vi "Atheros Tx CAL.vi"(6 "numAverages":u32, 7 "iMaxIteration":u32[](array[numeric]), 8 "error in (no error)":errorcluster, 9 "DebugInfo":bool, 10 "AllChainOn":bool, 11 "_hResourceContext":u32) -> (0 "error out":errorcluster, 2 "function return":bool, 3 "_hResourceContext out":u32)   [LabVIEW 2013, in "QCAWLAN_DLL.lvlib"]
doc: "QCA_DLL_Export bool Atheros_Tx_CAL (HANDLE _hResourceContext, bool AllChainOn, bool DebugInfo, unsigned int* iMaxIteration, unsigned int numAverages) ;"
uses:
  QCAWLAN_DLL.lvlib
  QCAWLAN_DLL.dll
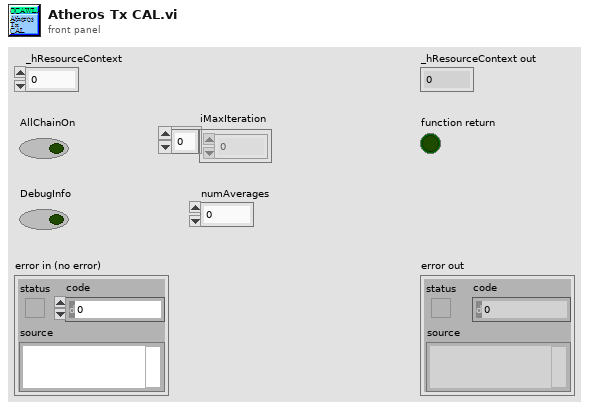
[diagram p1: front panel]
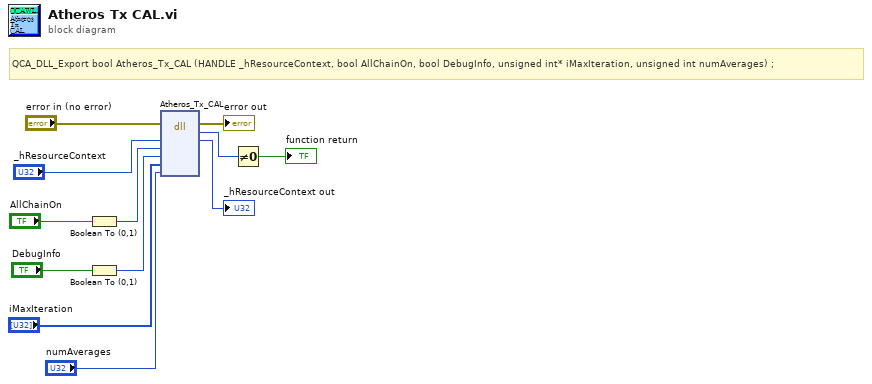
[diagram p0: block diagram]
diagram:
  # "QCA_DLL_Export bool Atheros_Tx_CAL (HANDLE _hResourceContext, bool AllChainOn, bool DebugInfo, unsigned int* iMaxIteration, unsigned int numAverages) ;"
  n1 = Boolean To (0,1)(Boolean="AllChainOn") -> (0, 1=w7:i16)
  n2 = Boolean To (0,1)(Boolean="DebugInfo") -> (0, 1=w5:i16)
  n3 = dll-call lib="C:/Connectivity Client - MIMO/PlugIn/QCAWLAN_DLL.*" fn="Atheros_Tx_CAL"(error in="error in (no error)", "_hResourceContext"="_hResourceContext", "AllChainOn"=w7, "DebugInfo"=w5, "iMaxIteration"="iMaxIteration", "numAverages"="numAverages") -> (error out=→"error out":errorcluster, "return type"=w11:u8, "_hResourceContext"=→"_hResourceContext out":u32)  [unwired: 6 in, 1 out]
  n4 = Not Equal To 0?(x=w11) -> (x != 0?=→"function return":bool)
